vi "Read name.vi"(11 "GUI in":refnum<class "GUI.lvclass">) -> (2 "name":string, 3 "GUI out":refnum<class "GUI.lvclass">)   [LabVIEW 2019, in "GUI.lvclass"]
uses:
  GUI.lvclass
  GUI.lvclass/GUI.ctl
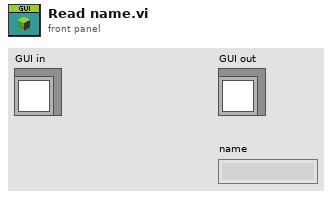
[diagram p1: front panel]
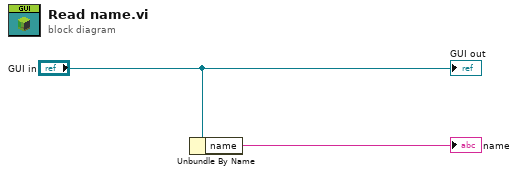
[diagram p0: block diagram]
diagram:
  n1 = Unbundle By Name("GUI in") -> ("name"=→"name":string)
  "GUI out" <- "GUI in"
